vi "gj.vi"() -> ()   [LabVIEW 2012]
panel:
  out "Array 7":dbl[][](array[numeric])
  out "Array 6":dbl[][](array[numeric])
  out "Array 3":dbl[][](array[numeric])
  out "Array 5":dbl[][](array[numeric])
  out "Array 4":dbl[][](array[numeric])
  out "Array 2":dbl[][](array[numeric])
  in  "Array":dbl[][](array[numeric])
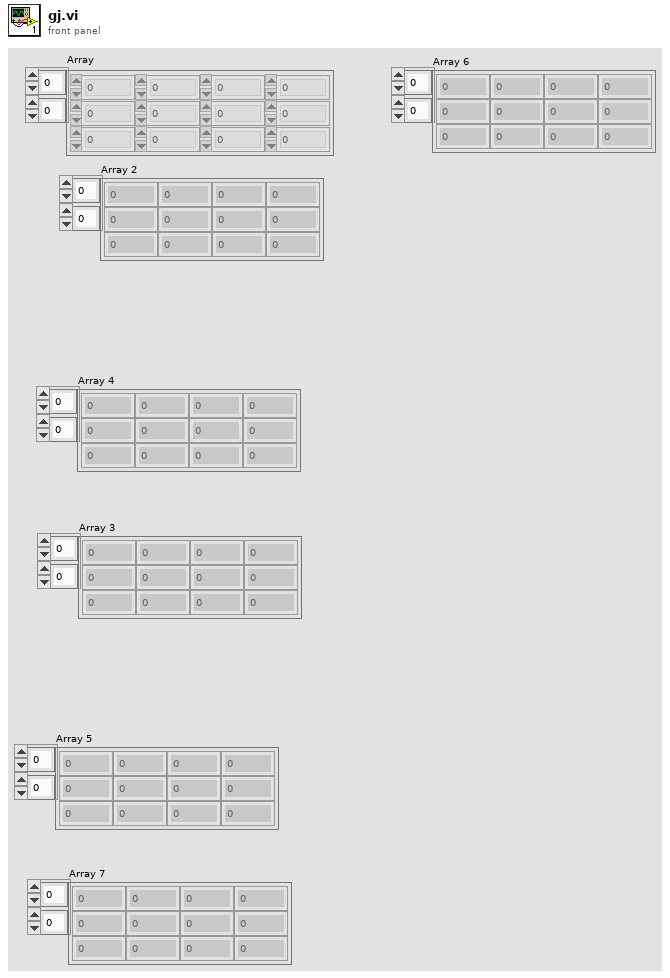
[diagram p1: front panel]
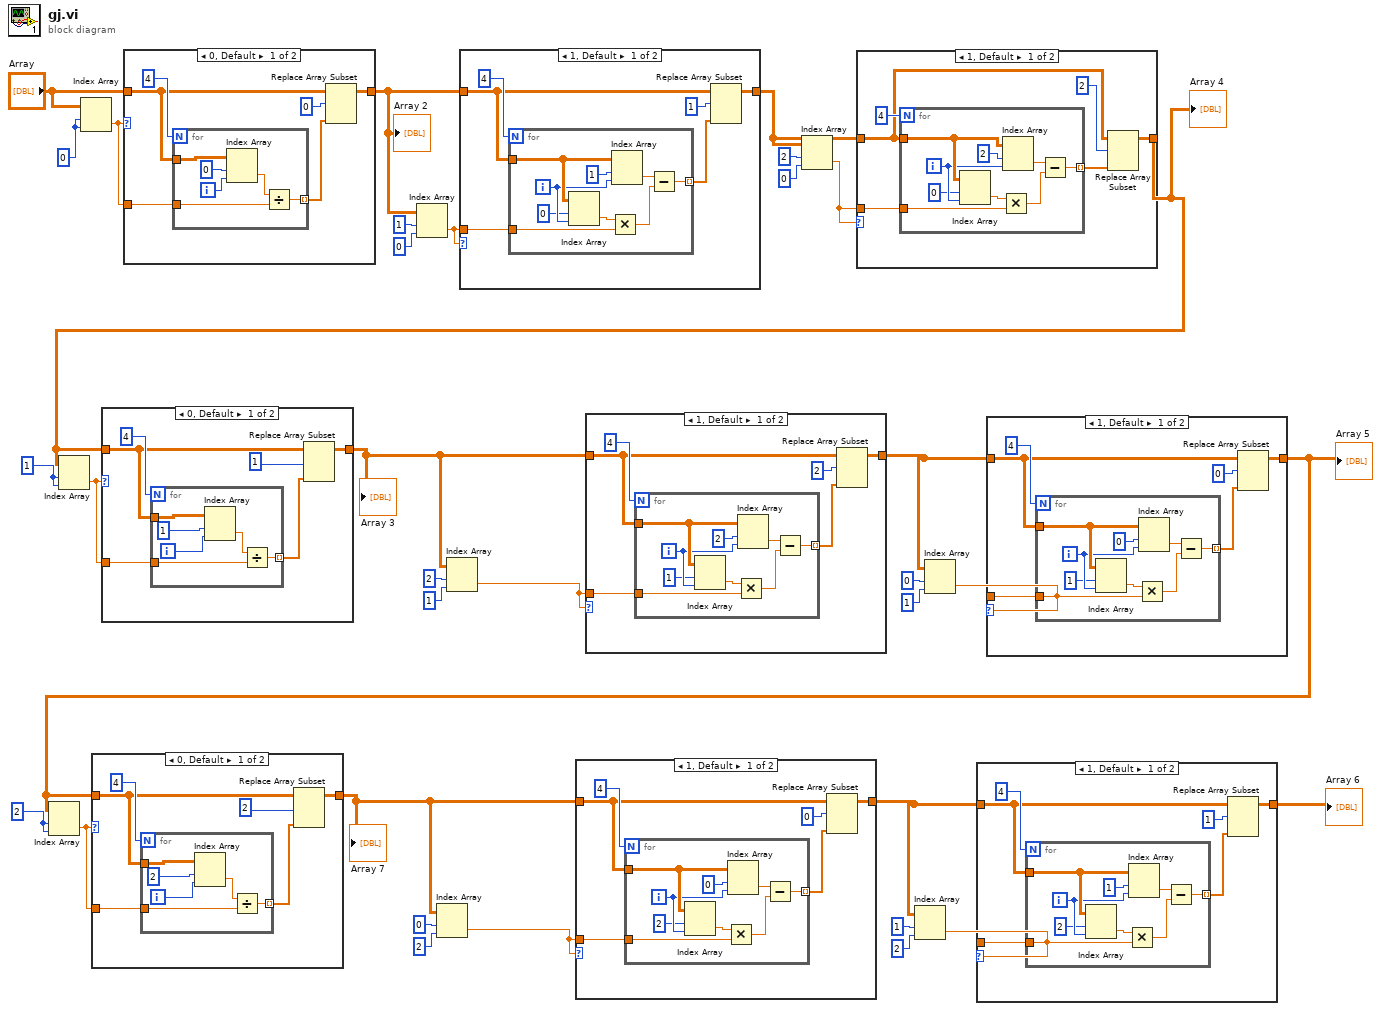
[diagram p0: block diagram]
diagram:
  w7 = 2 ("index (row)")
  w17 = 1 ("index (row)")
  w34 = 0 ("index (row)")
  n1 = Index Array(array="Array", index (row)=w34, index (col)=w34) -> (element=w33:dbl)
  n2 = case shown="0, Default" w33 {
    tunnel: w33 -> [w39 _]
    tunnel: "Array" -> [w37 w47]
    tunnel: [w36 w47] -> w29
    frame 0, Default {
      n3 = for {
        N: 4 -> [_]
        tunnel: w37 -> [w45]
        tunnel: w39 -> [w42]
        tunnel: [w43] -> w38 mode=indexing
        i -> [w44]
        n4 = Index Array(array=w45, index (row)=0 ("disabled index (row)"), index (col)=w44) -> (element=w41:dbl)
        n5 = Divide(x=w41, y=w42) -> (x/y=w43:dbl)
      }
      n6 = Replace Array Subset(array=w37, new element=w38, index (row)=0) -> (w36:dbl[][])  [unwired: 1 in]
    }
    frame 1 {
    }
  }
  "Array 2" <- w29
  n7 = Index Array(array=w29, index (row)=1, index (col)=0 ("disabled index (col)")) -> (element=w28:dbl)
  n8 = case shown="1, Default" w28 {
    tunnel: w29 -> [w50 w63]
    tunnel: w28 -> [w52 _]
    tunnel: [w48 w63] -> w24
    frame 1, Default {
      n9 = for {
        N: 4 -> [_]
        tunnel: w50 -> [w62]
        tunnel: w52 -> [w59]
        tunnel: [w54] -> w51 mode=indexing
        i -> [w61]
        n10 = Index Array(array=w62, index (row)=0 ("disabled index (row)"), index (col)=w61) -> (element=w60:dbl)
        n11 = Multiply(x=w60, y=w59) -> (x*y=w55:dbl)
        n12 = Index Array(array=w62, index (row)=1 ("disabled index (row)"), index (col)=w61) -> (element=w56:dbl)
        n13 = Subtract(x=w56, y=w55) -> (x-y=w54:dbl)
      }
      n14 = Replace Array Subset(array=w50, new element=w51, index (row)=1) -> (w48:dbl[][])  [unwired: 1 in]
    }
    frame 0 {
    }
  }
  n15 = Index Array(array=w24, index (row)=2, index (col)=0 ("disabled index (col)")) -> (element=w27:dbl)
  n16 = case shown="1, Default" w27 {
    tunnel: w24 -> [w66 w79]
    tunnel: w27 -> [w68 _]
    tunnel: [w64 w79] -> w18
    frame 1, Default {
      n17 = for {
        N: 4 -> [_]
        tunnel: w66 -> [w78]
        tunnel: w68 -> [w75]
        tunnel: [w70] -> w67 mode=indexing
        i -> [w77]
        n18 = Index Array(array=w78, index (row)=0 ("disabled index (row)"), index (col)=w77) -> (element=w76:dbl)
        n19 = Multiply(x=w76, y=w75) -> (x*y=w71:dbl)
        n20 = Index Array(array=w78, index (row)=2 ("disabled index (row)"), index (col)=w77) -> (element=w72:dbl)
        n21 = Subtract(x=w72, y=w71) -> (x-y=w70:dbl)
      }
      n22 = Replace Array Subset(array=w66, new element=w67, index (row)=2) -> (w64:dbl[][])  [unwired: 1 in]
    }
    frame 0 {
    }
  }
  "Array 4" <- w18
  n23 = Index Array(array=w18, index (row)=w17, index (col)=w17) -> (element=w19:dbl)
  n24 = case shown="0, Default" w19 {
    tunnel: w19 -> [w84 _]
    tunnel: w18 -> [w82 w92]
    tunnel: [w81 w92] -> w22
    frame 0, Default {
      n25 = for {
        N: 4 -> [_]
        tunnel: w82 -> [w90]
        tunnel: w84 -> [w88]
        tunnel: [w89] -> w83 mode=indexing
        i -> [w86]
        n26 = Index Array(array=w90, index (row)=1 ("disabled index (row)"), index (col)=w86) -> (element=w87:dbl)
        n27 = Divide(x=w87, y=w88) -> (x/y=w89:dbl)
      }
      n28 = Replace Array Subset(array=w82, new element=w83, index (row)=1) -> (w81:dbl[][])  [unwired: 1 in]
    }
    frame 1 {
    }
  }
  "Array 3" <- w22
  n29 = Index Array(array=w22, index (row)=2, index (col)=1 ("disabled index (col)")) -> (element=w23:dbl)
  n30 = case shown="1, Default" w23 {
    tunnel: w22 -> [w95 w108]
    tunnel: w23 -> [w97 _]
    tunnel: [w93 w108] -> w13
    frame 1, Default {
      n31 = for {
        N: 4 -> [_]
        tunnel: w95 -> [w107]
        tunnel: w97 -> [w104]
        tunnel: [w99] -> w96 mode=indexing
        i -> [w106]
        n32 = Index Array(array=w107, index (row)=1 ("disabled index (row)"), index (col)=w106) -> (element=w105:dbl)
        n33 = Multiply(x=w105, y=w104) -> (x*y=w100:dbl)
        n34 = Index Array(array=w107, index (row)=2 ("disabled index (row)"), index (col)=w106) -> (element=w101:dbl)
        n35 = Subtract(x=w101, y=w100) -> (x-y=w99:dbl)
      }
      n36 = Replace Array Subset(array=w95, new element=w96, index (row)=2) -> (w93:dbl[][])  [unwired: 1 in]
    }
    frame 0 {
    }
  }
  n37 = Index Array(array=w13, index (row)=0, index (col)=1 ("disabled index (col)")) -> (element=w14:dbl)
  n38 = case shown="1, Default" w14 {
    tunnel: w13 -> [w111 w124]
    tunnel: w14 -> [w113 _]
    tunnel: [w109 w124] -> w1
    frame 1, Default {
      n39 = for {
        N: 4 -> [_]
        tunnel: w111 -> [w123]
        tunnel: w113 -> [w120]
        tunnel: [w115] -> w112 mode=indexing
        i -> [w122]
        n40 = Index Array(array=w123, index (row)=1 ("disabled index (row)"), index (col)=w122) -> (element=w121:dbl)
        n41 = Multiply(x=w121, y=w120) -> (x*y=w116:dbl)
        n42 = Index Array(array=w123, index (row)=0 ("disabled index (row)"), index (col)=w122) -> (element=w117:dbl)
        n43 = Subtract(x=w117, y=w116) -> (x-y=w115:dbl)
      }
      n44 = Replace Array Subset(array=w111, new element=w112, index (row)=0) -> (w109:dbl[][])  [unwired: 1 in]
    }
    frame 0 {
    }
  }
  "Array 5" <- w1
  n45 = Index Array(array=w1, index (row)=w7, index (col)=w7) -> (element=w6:dbl)
  n46 = case shown="0, Default" w6 {
    tunnel: w6 -> [w129 _]
    tunnel: w1 -> [w127 w137]
    tunnel: [w126 w137] -> w3
    frame 0, Default {
      n47 = for {
        N: 4 -> [_]
        tunnel: w127 -> [w135]
        tunnel: w129 -> [w133]
        tunnel: [w134] -> w128 mode=indexing
        i -> [w131]
        n48 = Index Array(array=w135, index (row)=2 ("disabled index (row)"), index (col)=w131) -> (element=w132:dbl)
        n49 = Divide(x=w132, y=w133) -> (x/y=w134:dbl)
      }
      n50 = Replace Array Subset(array=w127, new element=w128, index (row)=2) -> (w126:dbl[][])  [unwired: 1 in]
    }
    frame 1 {
    }
  }
  "Array 7" <- w3
  n51 = Index Array(array=w3, index (row)=0, index (col)=2 ("disabled index (col)")) -> (element=w2:dbl)
  n52 = case shown="1, Default" w2 {
    tunnel: w3 -> [w140 w153]
    tunnel: w2 -> [w142 _]
    tunnel: [w138 w153] -> w11
    frame 1, Default {
      n53 = for {
        N: 4 -> [_]
        tunnel: w140 -> [w152]
        tunnel: w142 -> [w149]
        tunnel: [w144] -> w141 mode=indexing
        i -> [w151]
        n54 = Index Array(array=w152, index (row)=2 ("disabled index (row)"), index (col)=w151) -> (element=w150:dbl)
        n55 = Multiply(x=w150, y=w149) -> (x*y=w145:dbl)
        n56 = Index Array(array=w152, index (row)=0 ("disabled index (row)"), index (col)=w151) -> (element=w146:dbl)
        n57 = Subtract(x=w146, y=w145) -> (x-y=w144:dbl)
      }
      n58 = Replace Array Subset(array=w140, new element=w141, index (row)=0) -> (w138:dbl[][])  [unwired: 1 in]
    }
    frame 0 {
    }
  }
  n59 = Index Array(array=w11, index (row)=1, index (col)=2 ("disabled index (col)")) -> (element=w10:dbl)
  n60 = case shown="1, Default" w10 {
    tunnel: w11 -> [w156 w169]
    tunnel: w10 -> [w158 _]
    tunnel: [w154 w169] -> w12
    frame 1, Default {
      n61 = for {
        N: 4 -> [_]
        tunnel: w156 -> [w168]
        tunnel: w158 -> [w165]
        tunnel: [w160] -> w157 mode=indexing
        i -> [w167]
        n62 = Index Array(array=w168, index (row)=2 ("disabled index (row)"), index (col)=w167) -> (element=w166:dbl)
        n63 = Multiply(x=w166, y=w165) -> (x*y=w161:dbl)
        n64 = Index Array(array=w168, index (row)=1 ("disabled index (row)"), index (col)=w167) -> (element=w162:dbl)
        n65 = Subtract(x=w162, y=w161) -> (x-y=w160:dbl)
      }
      n66 = Replace Array Subset(array=w156, new element=w157, index (row)=1) -> (w154:dbl[][])  [unwired: 1 in]
    }
    frame 0 {
    }
  }
  "Array 6" <- w12
